vi "number_to_string.vi"() -> ()   [LabVIEW 2021]
panel:
  out "accuracy":dbl
  out "value":dbl
  out "resulting string":string
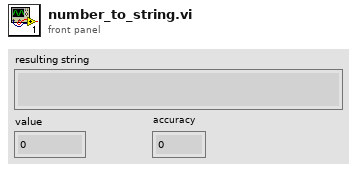
[diagram p1: front panel]
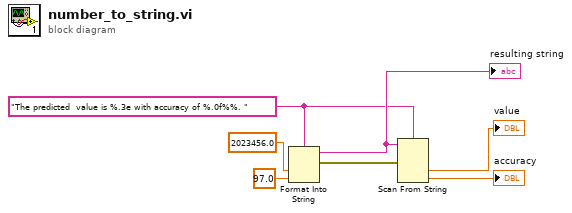
[diagram p0: block diagram]
diagram:
  w2 = "The predicted  value is %.3e with accuracy of %.0f%%. " ("format string")
  n1 = Format Into String "Format Into String"(format string=w2, 2023456.0 ("input 2"), 97.0 ("input 3")) -> (resulting string=w5:string, error out=w4:errorcluster)  [unwired: 2 in]
  "resulting string" <- w5
  n2 = Scan From String "Scan From String"(format string=w2, input string=w5, error in=w4) -> (output 1=→"value":dbl, output 2=→"accuracy":dbl)  [unwired: 3 in, 3 out]
